vi "setUp.vi"(8 "error in (no error)":errorcluster, 11 "reference in":refnum<class "Instrument Addon Common System Tests.lvclass">) -> (0 "error out":errorcluster, 3 "reference out":refnum<class "Instrument Addon Common System Tests.lvclass">)   [LabVIEW 2018, in "Instrument Addon Common System Tests.lvclass"]
doc: "setUp runs prior to the test method during test execution. Use this method to initialize any object data required by your tests."
uses:
  Instrument Addon Common System Tests.lvclass
  C:/Program Files (x86)/National Instruments/LabVIEW 2018/vi.lib/addons/_JKI Toolkits/VI Tester/TestCase.llb/TestCase.lvclass
  <vilib>/addons/_JKI Toolkits/VI Tester/TestCase.llb/TestCase.lvclass
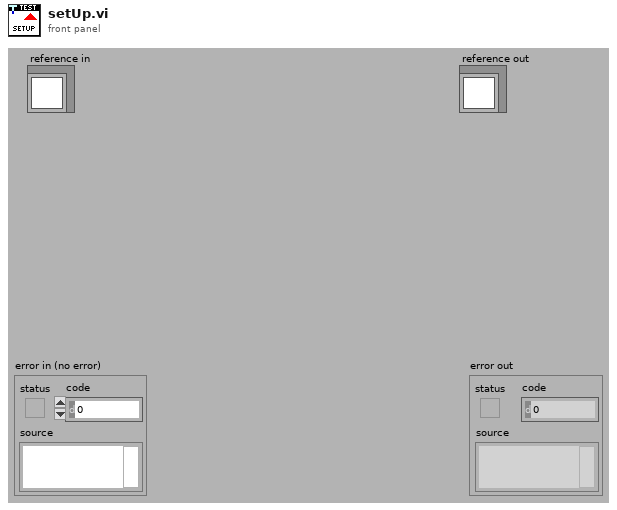
[diagram p1: front panel]
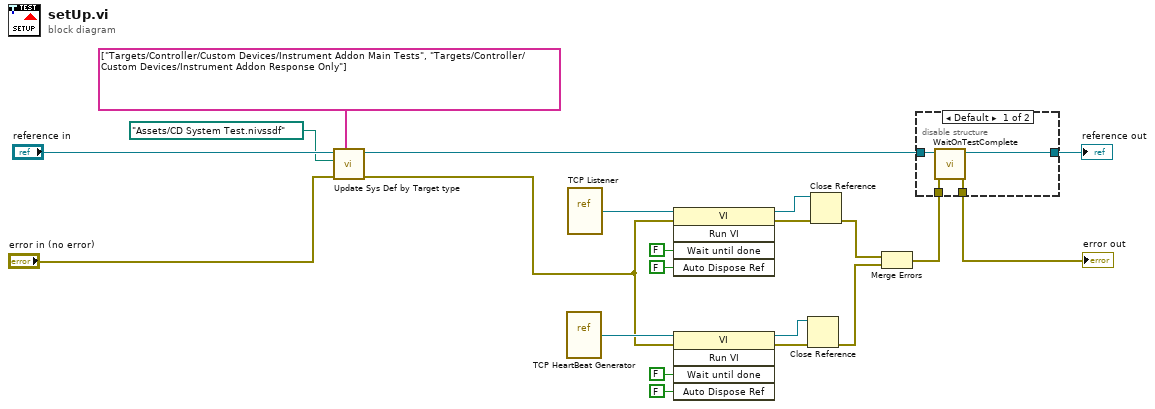
[diagram p0: block diagram]
diagram:
  n1 = call "Update Sys Def by Target type.vi"("nodepaths"=string[] ["Targets/Controller/Custom Devices/Instrument Addon Main Tests", "Targets/Controller/Custom Devices/Instrument Addon Response Only"], "error in (no error)"="error in (no error)", "Sys Def path:"=path "Assets/CD System Test.nivssdf", "reference in"="reference in") -> ("error out"=w4:errorcluster, "reference out"=w3:refnum<class "Instrument Addon Common System Tests.lvclass">)  [unwired: 6 in]
  n2 = vi-ref "TCP HeartBeat Generator.vi"() -> (w11:refnum<vi>)
  n3 = vi-ref "TCP Listener.vi"() -> (w19:refnum<vi>)
  n4 = invoke class="VI" method="Run VI"(reference=w19, error in=w4, "Wait until done"=FALSE ("Wait Until Done"), "Auto Dispose Ref"=FALSE ("Auto Dispose Reference")) -> (reference out=w18:refnum<vi>, error out=w17:errorcluster)  [unwired: 1 in, 3 out]
  n5 = invoke class="VI" method="Run VI"(reference=w11, error in=w4, "Wait until done"=FALSE ("Wait Until Done"), "Auto Dispose Ref"=FALSE ("Auto Dispose Reference")) -> (reference out=w9:refnum<vi>, error out=w8:errorcluster)  [unwired: 1 in, 3 out]
  n6 = Close Reference(reference=w9, error in (no error)=w8) -> (error out=w7:errorcluster)
  n7 = Close Reference(reference=w18, error in (no error)=w17) -> (error out=w16:errorcluster)
  n8 = Merge Errors(w16, w7) -> (w13:errorcluster)
  n9 = disable-structure shown="Default" {
    disable-tunnel: w13 -> [w25 w26]
    disable-tunnel: [w24 w26] -> w21
    disable-tunnel: [w23 w27] -> w20
    disable-tunnel: w3 -> [w22 w27]
    frame condition #0 (active) {
      n10 = call <vilib>:"WaitOnTestComplete.vi"("error in (no error)"=w25, "TestCase in"=w22) -> ("error out"=w24:errorcluster, "TestCase out"=w23:refnum<class "Instrument Addon Common System Tests.lvclass">)  [unwired: 8 in]
    }
    frame condition #1 {
    }
  }
  "error out" <- w21
  "reference out" <- w20
